vi "ReadMsgs.vi"(0 "reference in":refnum<class "MessageAMC.lvclass">, 11 "error in (no error)":errorcluster) -> (4 "reference out":refnum<class "MessageAMC.lvclass">, 6 "Array":T1[](array[typedef]), 15 "error out":errorcluster)   [LabVIEW 2019, in "MessageAMC.lvclass"]
uses:
  MessageAMC.lvclass
  MessageInterface_class/Message.ctl
  MessageAMC.lvclass/MessageAMC.ctl
  <vilib>/NI/AMC/Read Termination Message.vi
  <vilib>/NI/AMC/Create Single Message.vi
  <vilib>/NI/AMC/Globals.vi
  <vilib>/NI/AMC/AMC.lvlib
  MessageInterface_class/MessageInterface.lvclass
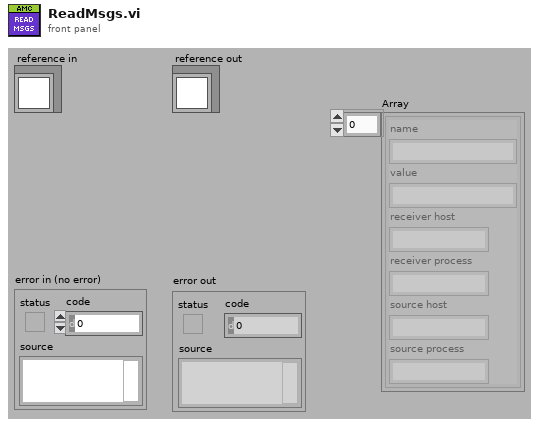
[diagram p1: front panel]
types:
  T1 = typedef "MessageInterface.lvclass/Message.ctl" = cluster{"name":string, "value":string, "receiver host":string, "receiver process":string, "source host":string, "source process":string}
  T2 = typedef "AMC.lvlib/Message Queue.ctl" = refnum<queue>
  T3 = typedef "AMC.lvlib/Message.ctl" = cluster{"name":string, "value":string, "attributes":T4, "receiver host":string, "receiver process":string, "source host":string, "source process":string, "priority message":bool, "acknowledge message":bool}
  T4 = typedef "Tools_KeyedArray.lvlib/KeyedArray.ctl" = cluster{"keys":string[], "values":string[]}
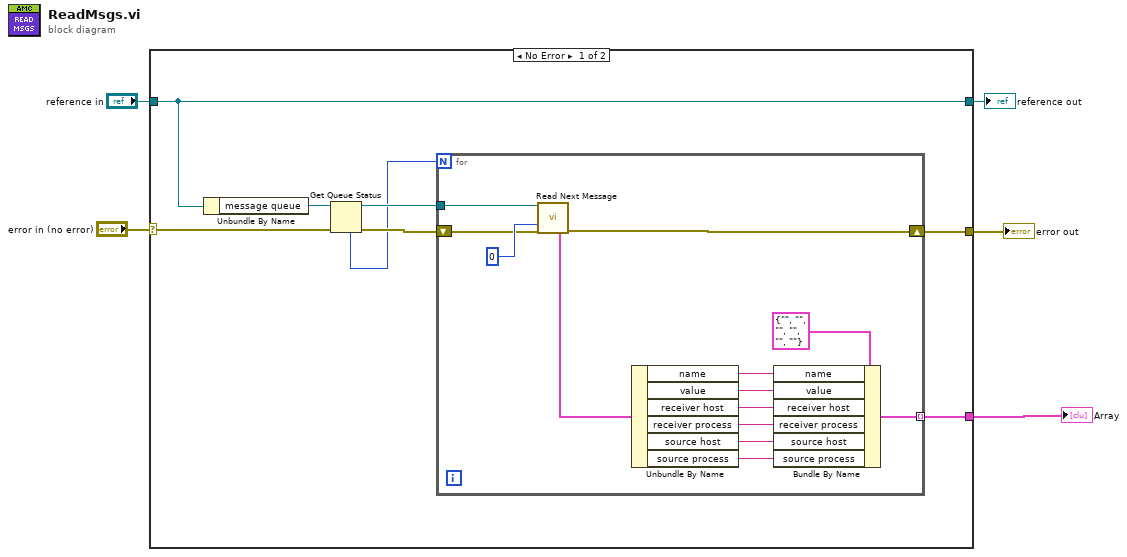
[diagram p0: block diagram]
diagram:
  n1 = case shown="No Error" "error in (no error)" {
    selector: "error in (no error)" -> [w8 w28]
    tunnel: [w12 w28] -> w4
    tunnel: [w13 w27] -> w2
    tunnel: "reference in" -> [w13 w27]
    tunnel: [w11 _] -> w1
    frame No Error {
      n2 = Unbundle By Name(w13) -> ("message queue"=w10:T2)
      n3 = Get Queue Status(queue=w10, error in (no error)=w8) -> (queue out=w9:T2, error out=w7:errorcluster, # elements in queue=w6:i32)  [unwired: 1 in, 5 out]
      n4 = for {
        N: w6 -> [_]
        tunnel: [w25] -> w11 mode=indexing
        tunnel: w9 -> [w15]
        shift-right: [w26] -> w12
        shift-left: w7 -> [w14]
        n5 = call <vilib>:"Read Next Message.vi"("message queue in"=w15, "timeout (1 ms)"=0, "error in"=w14) -> ("message"=w24:T3, "error out"=w26:errorcluster)  [unwired: 5 in, 6 out]
        n6 = Unbundle By Name(w24) -> ("name"=w23:string, "value"=w22:string, "receiver host"=w20:string, "receiver process"=w19:string, "source host"=w18:string, "source process"=w17:string)
        n7 = Bundle By Name(cluster=T1 {"name"="", "value"="", "receiver host"="", "receiver process"="", "source host"="", "source process"=""} ("message"), "name"=w23, "value"=w22, "receiver host"=w20, "receiver process"=w19, "source host"=w18, "source process"=w17) -> (w25:T1)
      }
    }
    frame Error {
    }
  }
  "error out" <- w4
  "reference out" <- w2
  "Array" <- w1
